vi "Get Marker.vi"(8 "Error In":errorcluster, 11 "Point":refnum<k24>) -> (0 "error out":errorcluster, 3 "new reference":refnum<k24>)   [LabVIEW 2014]
uses:
  C:/Robotic Systems/Products/AgFalcon/Software/Ground Station/Data/Mapping DLL/GMap.NET.WindowsForms.dll
  Data/Mapping DLL/GMap.NET.WindowsForms.dll
  C:/Robotic Systems/Products/AgFalcon/Software/Ground Station/Data/Mapping DLL/GMap.NET.Core.dll
  Data/Mapping DLL/GMap.NET.Core.dll
  System.Drawing
  MAVLink/Waypoint Controller/FGV/Methods/Get Waypoint type.vi
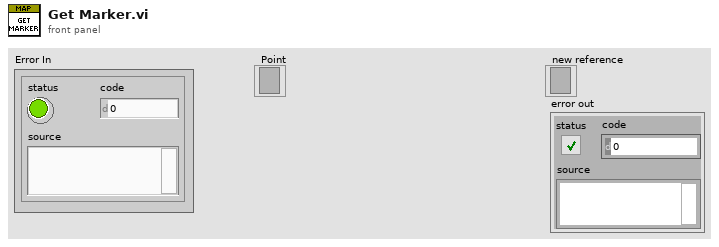
[diagram p1: front panel]
types:
  T1 = typedef "Waypoint Type.ctl" = enum16{"PASS-THROUGH", "INSPECT", "CIRCUMNAVIGATE"}
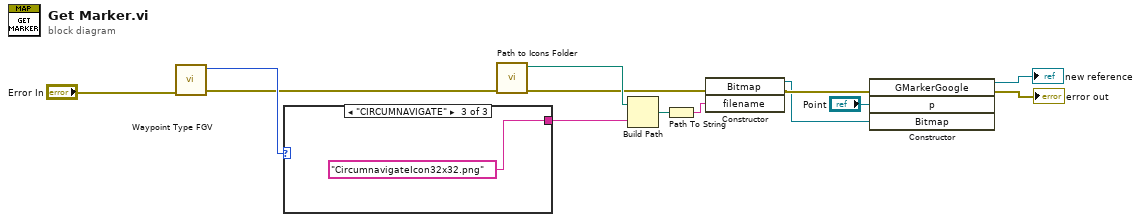
[diagram p0: block diagram]
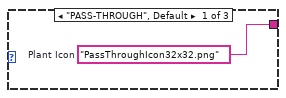
[diagram p2: hidden frame]
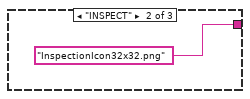
[diagram p3: hidden frame]
diagram:
  n1 = call-poly "Waypoint Type FGV.vi"("Error In"="Error In") -> ("Error Out"=w2:errorcluster, "Waypoint Type Out"=w12:T1)  [unwired: 9 in]
  n2 = case shown="\"CIRCUMNAVIGATE\"" w12 {
    tunnel: [w14 "InspectionIcon32x32.png" ("Plant Icon") "CircumnavigateIcon32x32.png" ("Plant Icon")] -> w1
    frame "PASS-THROUGH", Default {
      w14 = "PassThroughIcon32x32.png"  # Plant Icon
    }
    frame "INSPECT" {
    }
    frame "CIRCUMNAVIGATE" {
    }
  }
  n3 = call "Path to Icons Folder.vi"("Error In"=w2) -> ("Error Out"=w5:errorcluster, "Path to Icons Folder"=w7:path)  [unwired: 9 in]
  n4 = Build Path(base path=w7, name or relative path=w1) -> (appended path=w6:path)
  n5 = Path To String(path=w6) -> (string=w8:string)
  n6 = constructor class="Bitmap"(error in=w5, "filename"=w8) -> (reference out=w3:refnum<k24>, error out=w4:errorcluster)  [unwired: 2 in, 2 out]
  n7 = constructor class="GMarkerGoogle"(error in=w4, "p"="Point", "Bitmap"=w3) -> (reference out=→"new reference":refnum<k24>, error out=→"error out":errorcluster)  [unwired: 2 in, 3 out]
